vi "Control Panel.vi"(8 "error in (no error)":errorcluster, 11 "Fake cryostat in":refnum<class "Cryostat.lvclass">) -> (0 "error out":errorcluster, 3 "Fake cryostat out":refnum<class "Cryostat.lvclass">)   [LabVIEW 2017, in "Cryostat.lvclass"]
doc: "(Dynamic) A user-level application that simulates the physical front panel of the Instrument. Provide the user with buttons to manually control features of the instrument, and provide indicators of its current state."
uses:
  Cryostat.lvclass
  Cryostat.lvclass/Cryostat.ctl
  Utility Classes/Readable/Readable.lvclass
panel:
  in  "Query Control?":bool
  in  "Control On":bool
  out "In control mode?":bool
  in  "stop":bool
  in  "Set":bool
  in  "Read to Control":bool
  in  "Read":bool
  in  "Copy actual to set":bool
  in  "Populate fields with member data":bool
  out "Current set point":dbl
  in  "Desired set point":dbl
  out "Temperature B":dbl
  out "Temperature A":dbl
  # "Control Off"
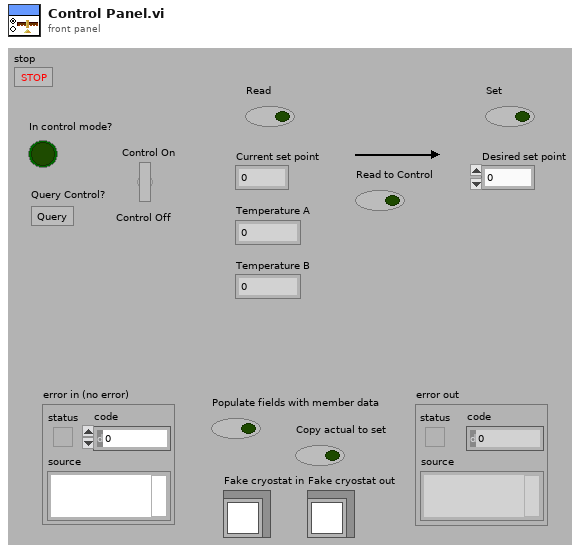
[diagram p1: front panel]
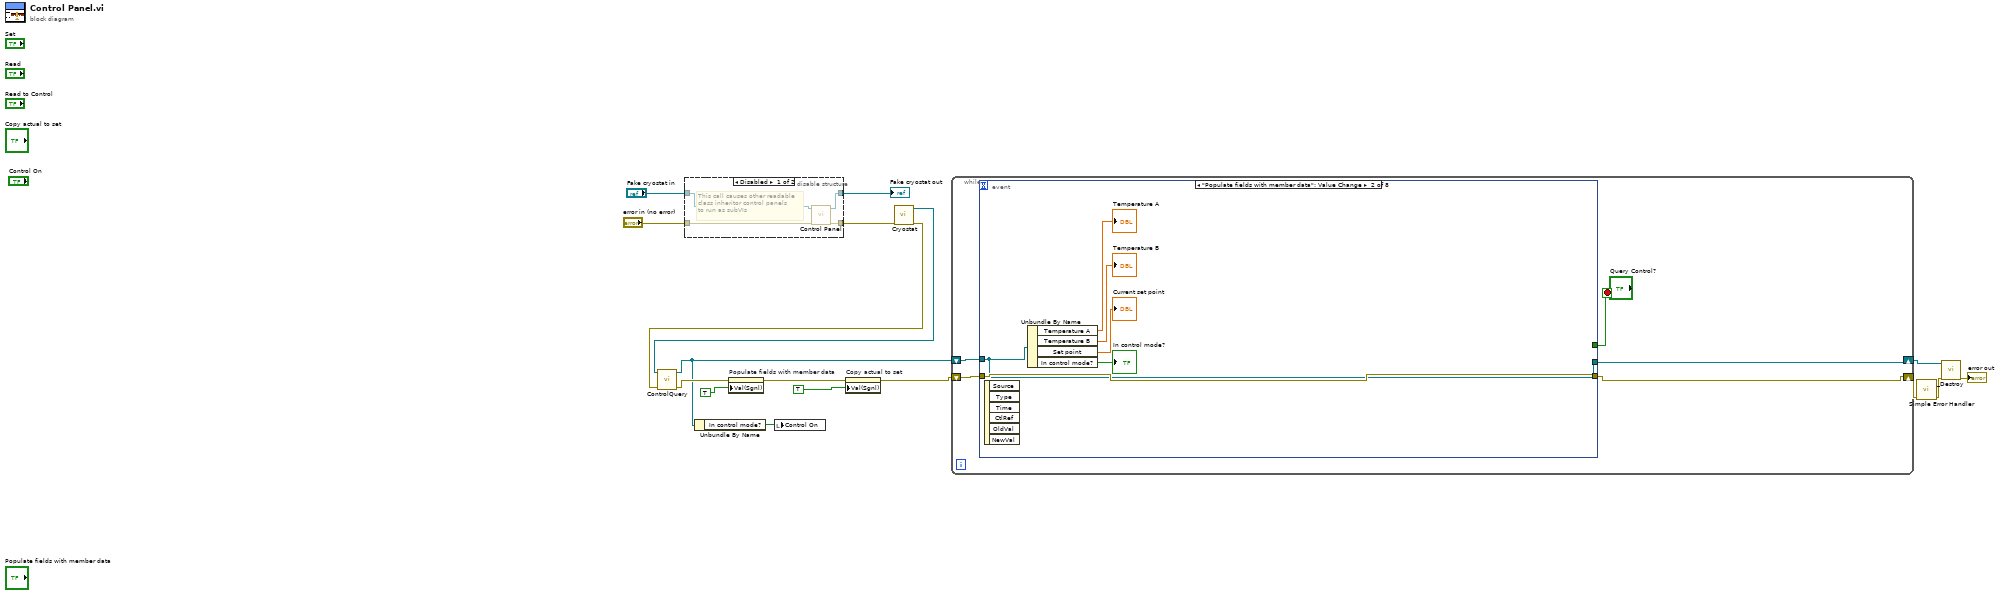
[diagram p0: block diagram]
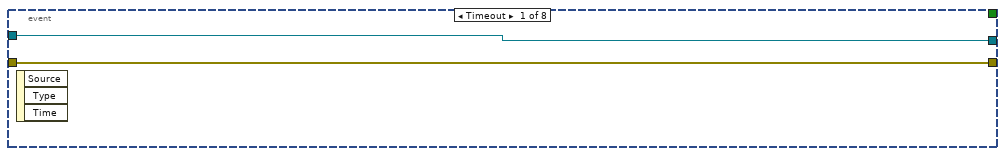
[diagram p3: hidden frame]
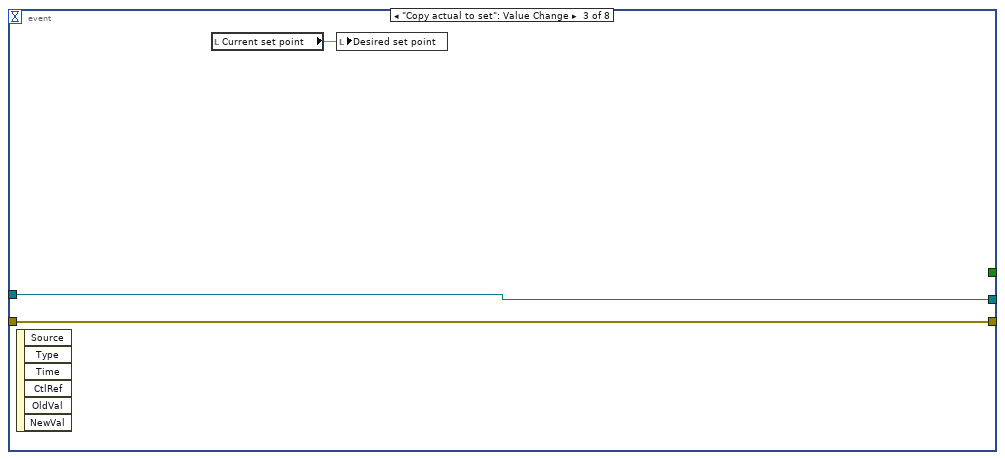
[diagram p4: hidden frame]
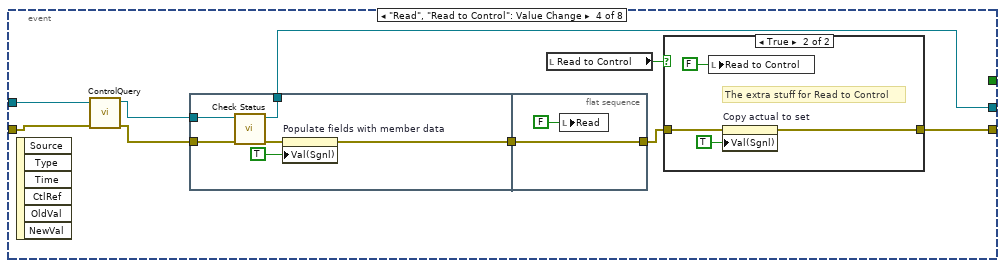
[diagram p5: hidden frame]
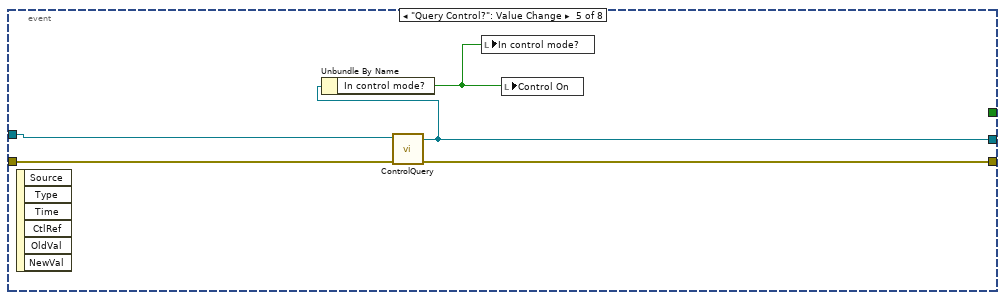
[diagram p7: hidden frame]
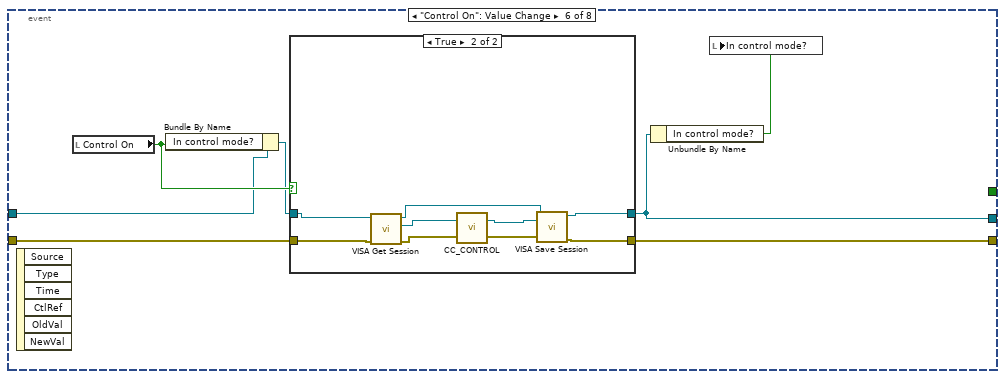
[diagram p8: hidden frame]
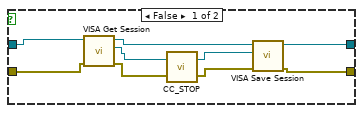
[diagram p9: hidden frame]
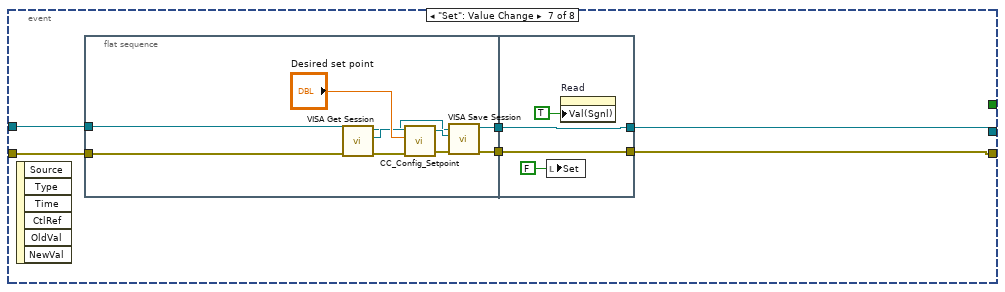
[diagram p10: hidden frame]
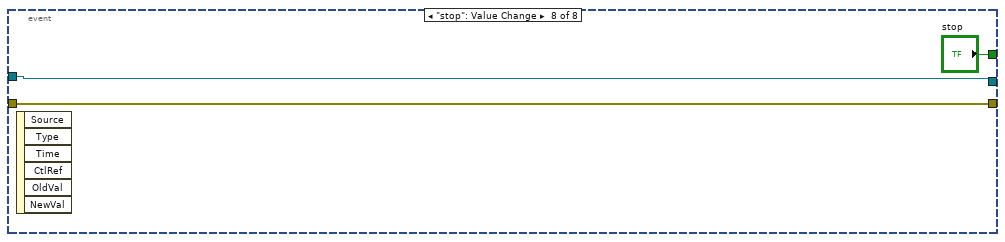
[diagram p11: hidden frame]
diagram:
  n1 = disable-structure shown="Disabled" {
    disable-tunnel: [w21 w23] -> w16
    disable-tunnel: "error in (no error)" -> [w20 w22]
    disable-tunnel: "Fake cryostat in" -> [w19 w23]
    disable-tunnel: [w18 w22] -> w15
    frame Disabled {
      # "This call causes other readable\nclass inheritor control panels\nto run as subVIs"
      n2 = call-parent "Control Panel.vi"("error in (no error)"=w20, "Instrument in"=w19) -> ("error out"=w18:errorcluster, "Instrument out"=w21:refnum<class "Cryostat.lvclass">)  [unwired: 8 out]
    }
    frame Enabled {
    }
  }
  "Fake cryostat out" <- w16
  n3 = call "Cryostat.vi"("error in (no error)"=w15) -> ("error out"=w7:errorcluster, "Cryostat out"=w8:refnum<class "Cryostat.lvclass">)  [unwired: 9 in]
  n4 = call "ControlQuery.vi"("error in (no error)"=w7, "Cryostat in"=w8) -> ("error out"=w6:errorcluster, "Cryostat out"=w2:refnum<class "Cryostat.lvclass">)  [unwired: 8 in]
  n5 = Unbundle By Name(w2) -> ("In control mode?"=w1:bool)
  n6 = property on="Populate fields with member data" class="Bool (strict)"(error in=w6, "Val(Sgnl)"=TRUE ("Value (Signaling)")) -> (error out=w11:errorcluster)  [unwired: 1 in, 1 out]
  n7 = local write "Control On"(w1) -> ()
  n8 = property on="Copy actual to set" class="Bool (strict)"(error in=w11, "Val(Sgnl)"=TRUE ("Value (Signaling)")) -> (error out=w9:errorcluster)  [unwired: 1 in, 1 out]
  n9 = while {
    shift-right: [w24] -> w4
    shift-left: w9 -> [w28]
    shift-right: [w25] -> w3
    shift-left: w2 -> [w26]
    stop <- w27 stop-if-true
    n10 = event shown="[1] \"Populate fields with member data\": Value Change" {
      selector: _ -> [_ _ _ _ _ _ _ _]
      dyn-events: _ -> [_ _ _ _ _ _ _ _]
      timeout: _ -> [_ _ _ _ _ _ _ _]
      tunnel: [w30 w35 w39 w41 w62 w67 w95 w113] -> w25
      tunnel: w26 -> [w30 w35 w39 w45 w64 w69 w96 w113]
      tunnel: [w29 w36 w38 w40 w65 w72 w94 w112] -> w24
      tunnel: w28 -> [w29 w36 w38 w44 w66 w73 w97 w112]
      tunnel: [_ _ _ _ _ _ _ "stop"] -> w27
      event Timeout {
        n11 = event-data() -> ()  [unwired: 1 in, 3 out]
      }
      event "Populate fields with member data": Value Change {
        n12 = event-data() -> ()  [unwired: 1 in, 6 out]
        n13 = Unbundle By Name(w35) -> ("Temperature A"=→"Temperature A":dbl, "Temperature B"=→"Temperature B":dbl, "Set point"=→"Current set point":dbl, "In control mode?"=→"In control mode?":bool)
      }
      event "Copy actual to set": Value Change {
        n14 = event-data() -> ()  [unwired: 1 in, 6 out]
        n15 = local read "Current set point"() -> (w37:dbl)
        n16 = local write "Desired set point"(w37) -> ()
      }
      event "Read", "Read to Control": Value Change {
        n17 = event-data() -> ()  [unwired: 1 in, 6 out]
        n18 = call "ControlQuery.vi"("error in (no error)"=w44, "Cryostat in"=w45) -> ("error out"=w43:errorcluster, "Cryostat out"=w42:refnum<class "Cryostat.lvclass">)  [unwired: 8 in]
        n19 = flat-sequence {
          tunnel: [w59] -> w41
          tunnel: [w56] -> w48
          tunnel: w43 -> [w55]
          tunnel: w42 -> [w54]
          tunnel: [w60] -> w46
          tunnel: w48 -> [w60]
          frame #0 {
            n20 = call-dynamic "Check Status.vi"("error in (no error)"=w55, "Cryostat in"=w54) -> ("error out"=w58:errorcluster, "Cryostat out"=w59:refnum<class "Cryostat.lvclass">)  [unwired: 8 out]
            n21 = property on="Populate fields with member data" class="Bool (strict)"(error in=w58, "Val(Sgnl)"=TRUE ("Value (Signaling)")) -> (error out=w56:errorcluster)  [unwired: 1 in, 1 out]
          }
          frame #1 {
            n22 = local write "Read"(FALSE ("Read")) -> ()
          }
        }
        n23 = local read "Read to Control"() -> (w47:bool)
        n24 = case shown="True" w47 {
          tunnel: w46 -> [w49 w51]
          tunnel: [w49 w50] -> w40
          frame False {
          }
          frame True {
            # "The extra stuff for Read to Control"
            n25 = local write "Read to Control"(FALSE ("Read to Control")) -> ()
            n26 = property on="Copy actual to set" class="Bool (strict)"(error in=w51, "Val(Sgnl)"=TRUE ("Value (Signaling)")) -> (error out=w50:errorcluster)  [unwired: 1 in, 1 out]
          }
        }
      }
      event "Query Control?": Value Change {
        n27 = event-data() -> ()  [unwired: 1 in, 6 out]
        n28 = call "ControlQuery.vi"("error in (no error)"=w66, "Cryostat in"=w64) -> ("error out"=w65:errorcluster, "Cryostat out"=w62:refnum<class "Cryostat.lvclass">)  [unwired: 8 in]
        n29 = Unbundle By Name(w62) -> ("In control mode?"=w63:bool)
        n30 = local write "In control mode?"(w63) -> ()
        n31 = local write "Control On"(w63) -> ()
      }
      event "Control On": Value Change {
        n32 = event-data() -> ()  [unwired: 1 in, 6 out]
        n33 = local read "Control On"() -> (w70:bool)
        n34 = Bundle By Name(cluster=w69, "In control mode?"=w70) -> (w68:refnum<class "Cryostat.lvclass">)
        n35 = case shown="True" w70 {
          tunnel: w68 -> [w82 w91]
          tunnel: [w80 w89] -> w67
          tunnel: w73 -> [w79 w88]
          tunnel: [w76 w85] -> w72
          frame False {
            n36 = call-dynamic "VISA Get Session.vi"("error in (no error)"=w79, "Instrument.lvclass in"=w82) -> ("error out"=w78:errorcluster, "VISA Resource Name"=w75:refnum<visa-resource-name>, "Instrument.lvclass out"=w81:refnum<class "Cryostat.lvclass">)  [unwired: 7 out]
            n37 = call "CC_STOP.vi"("error in (no error)"=w78, "VISA In"=w75) -> ("error out"=w77:errorcluster, "VISA Out"=w74:refnum<visa-resource-name>)
            n38 = call-dynamic "VISA Save Session.vi"("error in (no error)"=w77, "VISA Resource Name"=w74, "Instrument.lvclass in"=w81) -> ("error out"=w76:errorcluster, "Instrument.lvclass out"=w80:refnum<class "Cryostat.lvclass">)  [unwired: 7 out]
          }
          frame True {
            n39 = call-dynamic "VISA Get Session.vi"("error in (no error)"=w88, "Instrument.lvclass in"=w91) -> ("error out"=w87:errorcluster, "VISA Resource Name"=w84:refnum<visa-resource-name>, "Instrument.lvclass out"=w90:refnum<class "Cryostat.lvclass">)  [unwired: 7 out]
            n40 = call "CC_CONTROL.vi"("error in (no error)"=w87, "VISA In"=w84) -> ("error out"=w86:errorcluster, "VISA Out"=w83:refnum<visa-resource-name>)
            n41 = call-dynamic "VISA Save Session.vi"("error in (no error)"=w86, "VISA Resource Name"=w83, "Instrument.lvclass in"=w90) -> ("error out"=w85:errorcluster, "Instrument.lvclass out"=w89:refnum<class "Cryostat.lvclass">)  [unwired: 7 out]
          }
        }
        n42 = Unbundle By Name(w67) -> ("In control mode?"=w71:bool)
        n43 = local write "In control mode?"(w71) -> ()
      }
      event "Set": Value Change {
        n44 = event-data() -> ()  [unwired: 1 in, 6 out]
        n45 = flat-sequence {
          tunnel: w97 -> [w107]
          tunnel: w96 -> [w103]
          tunnel: [w100] -> w93
          tunnel: [w99] -> w92
          tunnel: [w110] -> w94
          tunnel: [w111] -> w95
          tunnel: w93 -> [w111]
          tunnel: w92 -> [w110]
          frame #0 {
            n46 = call-dynamic "VISA Get Session.vi"("error in (no error)"=w107, "Instrument.lvclass in"=w103) -> ("error out"=w104:errorcluster, "VISA Resource Name"=w105:refnum<visa-resource-name>, "Instrument.lvclass out"=w98:refnum<class "Cryostat.lvclass">)  [unwired: 7 out]
            n47 = call "CC_Config_Setpoint.vi"("error in (no error)"=w104, "Set Point"="Desired set point", "VISA In"=w105) -> ("error out"=w102:errorcluster, "VISA Out"=w101:refnum<visa-resource-name>)  [unwired: 1 in, 1 out]
            n48 = call-dynamic "VISA Save Session.vi"("error in (no error)"=w102, "VISA Resource Name"=w101, "Instrument.lvclass in"=w98) -> ("error out"=w99:errorcluster, "Instrument.lvclass out"=w100:refnum<class "Cryostat.lvclass">)  [unwired: 7 out]
          }
          frame #1 {
            n49 = local write "Set"(FALSE ("Set")) -> ()
            n50 = property on="Read" class="Bool (strict)"("Val(Sgnl)"=TRUE ("Value (Signaling)")) -> ()  [unwired: 2 in, 2 out]
          }
        }
      }
      event "stop": Value Change {
        n51 = event-data() -> ()  [unwired: 1 in, 6 out]
      }
    }
  }
  n52 = call <vilib>:"Simple Error Handler.vi"("error in (no error)"=w4) -> ("error out"=w14:errorcluster)  [unwired: 1 in, 7 out]
  n53 = call-dynamic "_Destroy.vi"("error in (no error)"=w14, "Instrument in"=w3) -> ("error out"=→"error out":errorcluster)  [unwired: 9 out]
